vi "draw flatten jpg to pic ctrl.vi"(8 "error in (no error)":errorcluster, 11 "path to JPEG file":path) -> (0 "error out":errorcluster, 1 "Picture":picture)   [LabVIEW 2017]
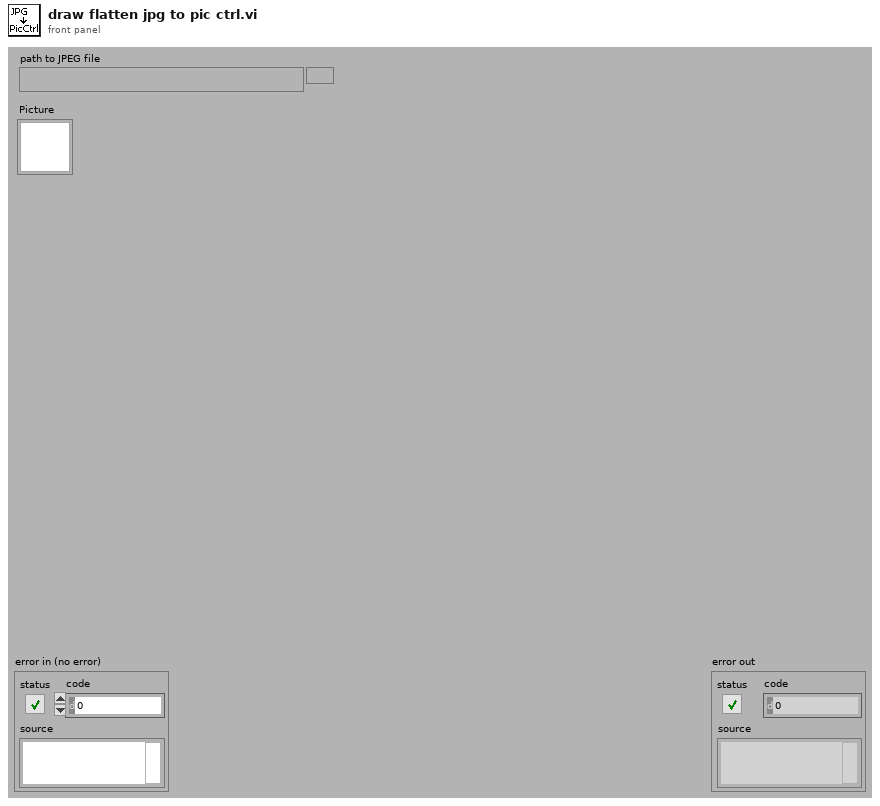
[diagram p1: front panel]
types:
  T1 = cluster{"left":i16, "top":i16, "right":i16, "bottom":i16}
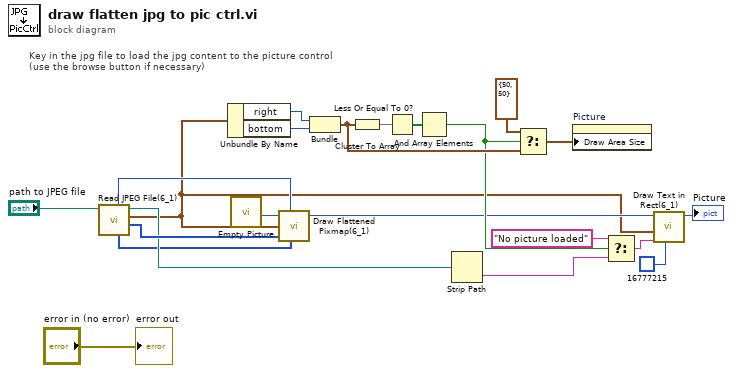
[diagram p0: block diagram]
diagram:
  # "Key in the jpg file to load the jpg content to the picture control\n(use the browse button if necessary)"
  n1 = call <vilib>:"Read JPEG File(6_1).vi"("path to JPEG file"="path to JPEG file") -> ("flattened image data"=w21:u8[], "rect"=w6:T1, "path"=w8:path, "colorTable"=w5:u32[], "depth"=w20:u8)  [unwired: 5 in, 1 out]
  n2 = Unbundle By Name(w6) -> ("right"=w17:i16, "bottom"=w18:i16)
  n3 = call "Empty Picture"() -> ("empty picture"=w19:picture)
  n4 = call <vilib>:"Draw Flattened Pixmap(6_1).vi"("picture"=w19, "bit depth(8)"=w20, "rect"=w6, "flattened pixmap data"=w21, "color table"=w5) -> ("new picture"=w9:picture)  [unwired: 4 in]
  n5 = Bundle("right"=w17, "bottom"=w18) -> (w14:cluster{"right":i16, "bottom":i16})  [unwired: 1 in]
  n6 = Cluster To Array(cluster=w14) -> (array=w16:i16[])
  n7 = Less Or Equal To 0?(x=w16) -> (x <= 0?=w15:bool[])
  n8 = And Array Elements(Boolean array=w15) -> (logical AND=w13:bool)
  n9 = Strip Path(path=w8) -> (name=w7:string)  [unwired: 1 out]
  n10 = Select(t=cluster{"Width":u32, "Height":u32} {"Width"=50, "Height"=50} ("Draw Area Size"), s=w13, f=w14) -> (s? t:f=w3:cluster{"Width":u32, "Height":u32})
  n11 = property on="Picture" class="Pict"("Draw Area Size"=w3) -> ()  [unwired: 2 in, 2 out]
  n12 = Select(t="No picture loaded", s=w13, f=w7) -> (s? t:f=w11:string)
  n13 = call <vilib>:"Draw Text in Rect(6_1).vi"("text color(black)"=u32 16777215, "text"=w11, "rect"=w6, "picture"=w9) -> ("new picture"=→"Picture":picture)  [unwired: 7 in]
  "error out" <- "error in (no error)"
